vi "ListaKto_new.vi"(8 "error in (no error)":errorcluster, 10 "Jsonconfig":string) -> (0 "error out":errorcluster, 2 "Array":i32[](array[numeric]), 3 "Array 2":string[](array[string]))   [LabVIEW 2017]
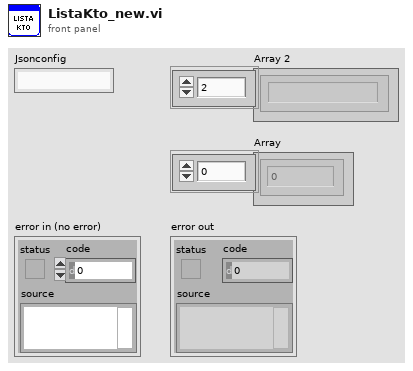
[diagram p1: front panel]
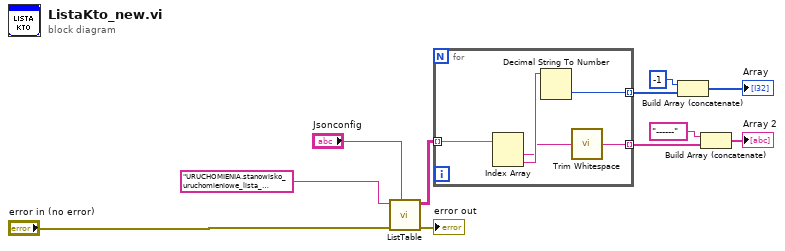
[diagram p0: block diagram]
diagram:
  n1 = call "ListTable.vi"("Jsonconfig"="Jsonconfig", "error in (no error)"="error in (no error)", "table"="URUCHOMIENIA.stanowisko_uruchomieniowe_lista_uruchamiajacych") -> ("error out"=→"error out":errorcluster, "data"=w4:string[][])  [unwired: 7 in]
  n2 = for {
    tunnel: w4 -> [w16] mode=indexing
    tunnel: [w12] -> w8 mode=indexing
    tunnel: [w15] -> w9 mode=indexing
    n3 = Index Array(array=w16) -> (element #1=w13:string, element #2=w14:string)  [unwired: 2 in]
    n4 = Decimal String To Number(string=w14) -> (number=w15:i32)  [unwired: 2 in, 1 out]
    n5 = call <vilib>:"Trim Whitespace.vi"("string"=w13) -> ("trimmed string"=w12:string)  [unwired: 1 in]
  }
  n6 = Build Array (concatenate)(-1 ("number"), w9) -> (→"Array":i32[])
  n7 = Build Array (concatenate)("------", w8) -> (→"Array 2":string[])
